vi "Create Policy.vi"(8 "error in (no error)":errorcluster, 9 "Policy JSON":string, 10 "Name":string, 11 "IoT Session in":refnum<class "IoT Session.lvclass">) -> (0 "error out":errorcluster, 3 "IoT Session out":refnum<class "IoT Session.lvclass">)   [LabVIEW 2015, in "NI_AWS_IoT.lvlib" / "IoT Session.lvclass"]
uses:
  IoT Session.lvclass
  Core/HTTP Request/Valid String Specification.ctl
  Core/HTTP Request/Request Options.ctl
  Core/HTTP Request/Name Value Pair.ctl
  Core/HTTP Request/Region handling.ctl
  Core/HTTP Request/URL formatting.ctl
  Core/HTTP Request/HTTP Request.lvclass
  JSON Parsing/NI_JSON Parsing.lvlib
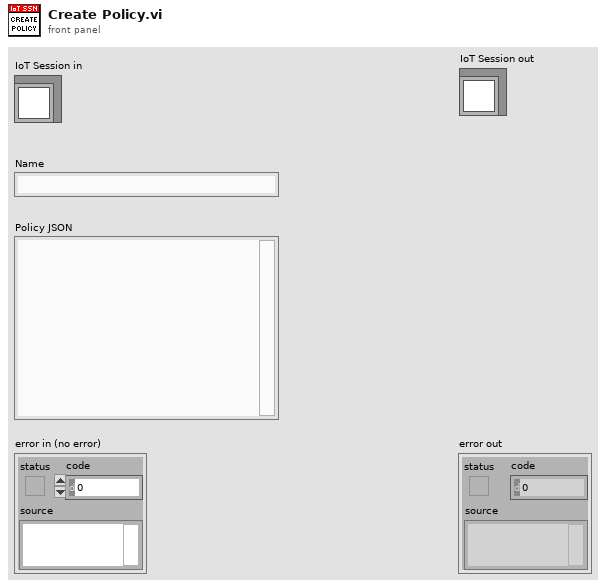
[diagram p1: front panel]
types:
  T1 = typedef "NI_AWS_Core.lvlib/HTTP Request.lvclass/Valid String Specification.ctl" = enum16{"none", "only [alphanumeric][-][_]", "only [alphanumeric][-][_][space]", "phone number +1xxxyyyzzzz", "Regular Expression"}
  T2 = typedef "NI_AWS_Core.lvlib/HTTP Request.lvclass/Name Value Pair.ctl" = cluster{"name":string, "value":string}
  T3 = typedef "NI_AWS_Core.lvlib/HTTP Request.lvclass/Request Options.ctl" = cluster{"request headers":T2[], "request parameters":T2[], "request body":string, "region handling":T4, "URL formatting":T5}
  T4 = typedef "NI_AWS_Core.lvlib/HTTP Request.lvclass/Region handling.ctl" = enum16{"use region everywhere", "use region (authentication only)", "use region (URL only)", "ignore region everwhere"}
  T5 = typedef "NI_AWS_Core.lvlib/HTTP Request.lvclass/URL formatting.ctl" = enum16{"region-", "region."}
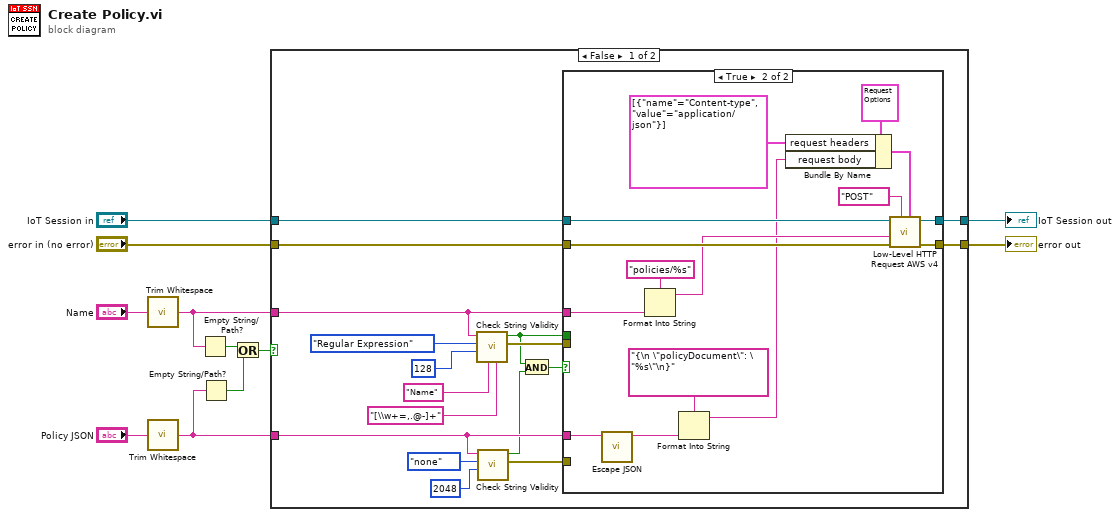
[diagram p0: block diagram]
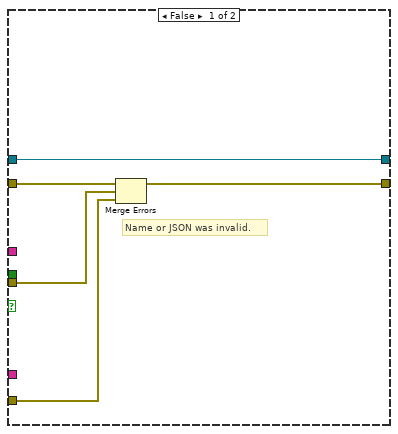
[diagram p2: hidden frame]
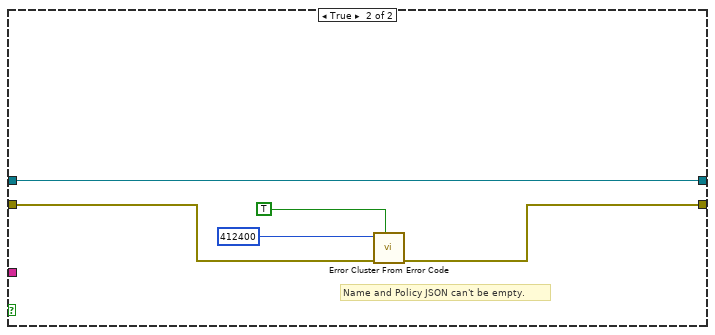
[diagram p3: hidden frame]
diagram:
  n1 = call <vilib>:"Trim Whitespace.vi"("string"="Name") -> ("trimmed string"=w5:string)  [unwired: 1 in]
  n2 = call <vilib>:"Trim Whitespace.vi"("string"="Policy JSON") -> ("trimmed string"=w4:string)  [unwired: 1 in]
  n3 = Empty String/Path?(string/path=w5) -> (empty?=w3:bool)
  n4 = Empty String/Path?(string/path=w4) -> (empty?=w2:bool)
  n5 = Or(x=w3, y=w2) -> (x .or. y?=w1:bool)
  n6 = case shown="False" w1 {
    tunnel: "error in (no error)" -> [w28 w53]
    tunnel: [w27 w52] -> w10
    tunnel: [w26 w50] -> w9
    tunnel: w4 -> [w15 _]
    tunnel: "IoT Session in" -> [w21 w50]
    tunnel: w5 -> [w18 _]
    frame False {
      n7 = call "Check String Validity.vi"("Regular Expression"="[\\w+=,.@-]+", "String Name for Error"="Name", "Max Characters"=128, "Valid String Specification"=Valid_String_Specification."Regular Expression", "String"=w18) -> ("string error"=w22:errorcluster, "Valid"=w19:bool)  [unwired: 5 in]
      n8 = call "Check String Validity.vi"("Max Characters"=2048, "Valid String Specification"=Valid_String_Specification."none", "String"=w15) -> ("string error"=w14:errorcluster, "Valid"=w13:bool)  [unwired: 7 in]
      n9 = And(x=w19, y=w13) -> (x .and. y?=w12:bool)
      n10 = case shown="True" w12 {
        tunnel: w28 -> [w33 w48]
        tunnel: [w32 w47] -> w27
        tunnel: [w30 w46] -> w26
        tunnel: w18 -> [_ w42]
        tunnel: w22 -> [w31 _]
        tunnel: w21 -> [w30 w38]
        tunnel: w15 -> [_ w35]
        tunnel: w14 -> [w29 _]
        tunnel: w19 -> [_ _]
        frame False {
          # "Name or JSON was invalid."
          n11 = Merge Errors(w33, w31, w29) -> (w32:errorcluster)
        }
        frame True {
          n12 = call "Escape JSON.vi"("JSON"=w35) -> ("Escaped JSON"=w34:string)  [unwired: 10 in]
          n13 = Format Into String(format string="policies/%s", w42) -> (resulting string=w43:string)  [unwired: 2 in, 1 out]
          n14 = Format Into String(format string="{\n \"policyDocument\": \"%s\"\n}", w34) -> (resulting string=w36:string)  [unwired: 2 in, 1 out]
          n15 = Bundle By Name(cluster=T3 {"request headers"=[], "request parameters"=[], "request body"="", "region handling"=enum."use region everywhere", "URL formatting"=enum."region."} ("Request Options"), "request headers"=T2[] [{"name"="Content-type", "value"="application/json"}], "request body"=w36) -> (w40:T3)
          n16 = call "Low-Level HTTP Request AWS v4.vi"("Request Options"=w40, "HTTP-Verb"="POST", "error in (no error)"=w48, "URL Suffix"=w43, "AWS Core in"=w38) -> ("error out"=w47:errorcluster, "AWS Core out"=w46:refnum<class "IoT Session.lvclass">)  [unwired: 3 in, 2 out]
        }
      }
    }
    frame True {
      # "Name and Policy JSON can't be empty."
      n17 = call <vilib>:"Error Cluster From Error Code.vi"("show call chain? (False)"=TRUE, "error in (no error)"=w53, "error code (0)"=412400) -> ("error out"=w52:errorcluster)  [unwired: 6 in]
    }
  }
  "error out" <- w10
  "IoT Session out" <- w9
